vi "System Data Format.vi"(8 "error in (no error)":errorcluster, 9 "Data Length (6)":i32=6, 10 "Format (ASCII)":i32(ring) items=["ASCII", "Real", "Binary", "Hexadecimal", "Octal"], 11 "VISA resource name":refnum<visa-resource-name>) -> (0 "error out":errorcluster, 3 "VISA resource name out":refnum<visa-resource-name>)   [LabVIEW 2015, in "Rohde&Schwarz CMXP Base.lvlib"]
doc: "Selects the format for numeric data transferred to and from the R&SCMX500, for example query results.\n\nAttribute:\n-\n\nRemote-control command:\nFORMat:BASE[:DATA]"
uses:
  <instrlib>/Rohde&Schwarz CMXP Base/Rohde&Schwarz CMXP Base.lvlib
  <instrlib>/Rohde&Schwarz CMXP Base/Private/rsidr_core.llb/rsidr_core.lvlib
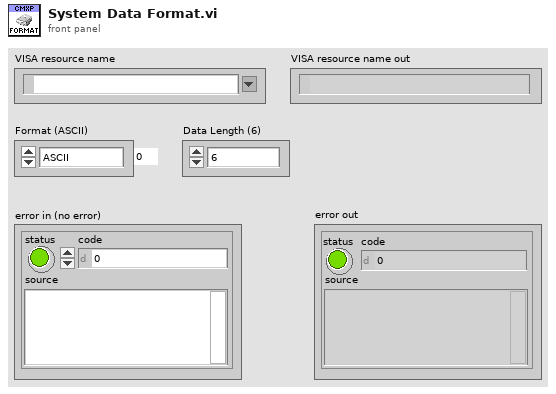
[diagram p1: front panel]
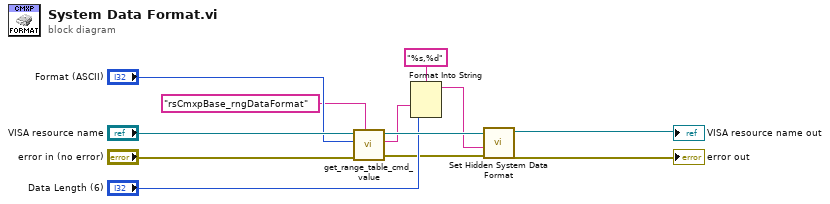
[diagram p0: block diagram]
diagram:
  n1 = call <instrlib>:"get_range_table_cmd_value.vi"("Range Table ID in"="rsCmxpBase_rngDataFormat", "error in"="error in (no error)", "Input Int32 value"="Format (ASCII)", "VISA resource name"="VISA resource name") -> ("error out"=w3:errorcluster, "Cmd value out"=w1:string, "VISA resource name out"=w5:refnum<visa-resource-name>)  [unwired: 5 in]
  n2 = Format Into String(format string="%s,%d", w1, "Data Length (6)") -> (resulting string=w2:string)  [unwired: 2 in, 1 out]
  n3 = call "Set Hidden System Data Format"("error in (no error)"=w3, "Hidden System Data Format ()"=w2, "instrument handle"=w5) -> ("error out"=→"error out":errorcluster, "instrument handle out"=→"VISA resource name out":refnum<visa-resource-name>)  [unwired: 7 in]
